vi "Valid Measurement Service Name.vi"(8 "error in":errorcluster, 11 "requested plugin name":string) -> (0 "error out":errorcluster, 3 "valid name?":bool)   [LabVIEW 2021, in "Migrator.lvlib"]
uses:
  Migrator.lvlib
  48953c88-0603-4c13-ba6a-df914321b09e.vi
  <vilib>/Comparison/Equal/Equal Functor/Equal Functor.lvclass
  Measurement Plugin Generator/_Editor/MeasurementService Editor.lvlib
panel:
  out "control chars":string
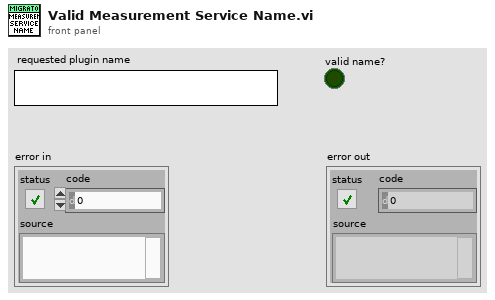
[diagram p1: front panel]
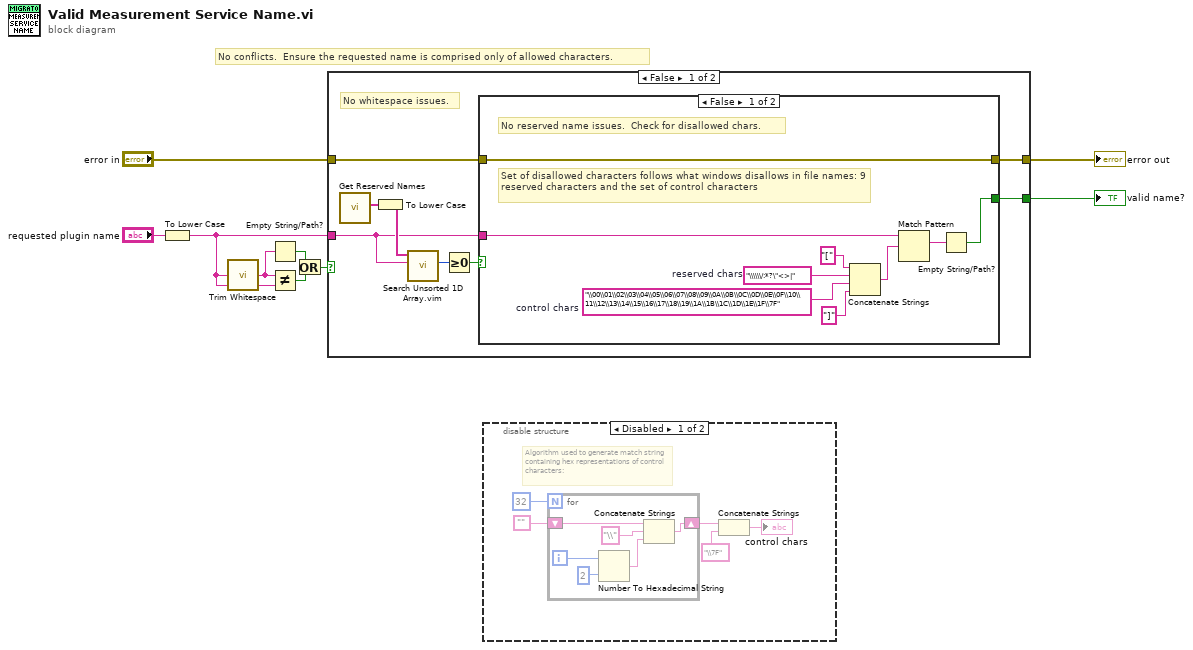
[diagram p0: block diagram]
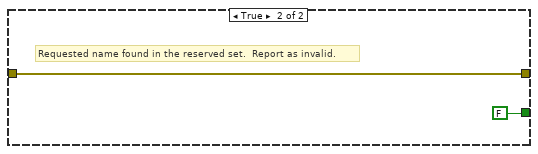
[diagram p2: hidden frame]
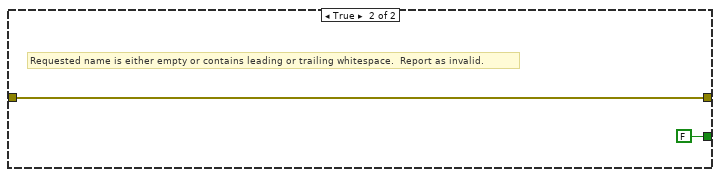
[diagram p3: hidden frame]
diagram:
  # "No conflicts.  Ensure the requested name is comprised only of allowed characters."
  n1 = To Lower Case(string="requested plugin name") -> (all lower case string=w5:string)
  n2 = call <vilib>:"Trim Whitespace.vi"("string"=w5) -> ("trimmed string"=w4:string)  [unwired: 1 in]
  n3 = Empty String/Path?(string/path=w4) -> (empty?=w2:bool)
  n4 = Not Equal?(x=w4, y=w5) -> (x != y?=w3:bool)
  n5 = Or(x=w2, y=w3) -> (x .or. y?=w1:bool)
  n6 = case shown="False" w1 {
    tunnel: w5 -> [w13 _]
    tunnel: "error in" -> [w17 w30]
    tunnel: [w16 w30] -> w7
    tunnel: [w10 FALSE ("Error if not Found (T)")] -> w6
    frame False {
      # "No whitespace issues."
      n7 = call "Get Reserved Names.vi"() -> ("reserved names"=w15:string[])  [unwired: 11 in]
      n8 = To Lower Case(string=w15) -> (all lower case string=w14:string[])
      n9 = call "Search Unsorted 1D Array.vim"("element"=w13, "unsorted 1D array"=w14) -> ("index of element"=w12:i32)  [unwired: 9 in]
      n10 = Greater Or Equal To 0?(x=w12) -> (x >= 0?=w11:bool)
      n11 = case shown="False" w11 {
        tunnel: w13 -> [w25 _]
        tunnel: w17 -> [w26 w28]
        tunnel: [w26 w28] -> w16
        tunnel: [w23 FALSE ("Error if not Found (T)")] -> w10
        frame False {
          w18 = "\\00\\01\\02\\03\\04\\05\\06\\07\\08\\09\\0A\\0B\\0C\\0D\\0E\\0F\\10\\11\\12\\13\\14\\15\\16\\17\\18\\19\\1A\\1B\\1C\\1D\\1E\\1F\\7F"  # control chars
          w22 = "\\\\\\/:*?\"<>|"  # reserved chars
          # "Set of disallowed characters follows what windows disallows in file names: 9 reserved characters and the set of control characters"
          # "No reserved name issues.  Check for disallowed chars."
          n12 = Concatenate Strings("[" ("string"), w22, w18, "]" ("string")) -> (w19:string)
          n13 = Match Pattern(string=w25, regular expression=w19) -> (match substring=w24:string)  [unwired: 1 in, 3 out]
          n14 = Empty String/Path?(string/path=w24) -> (empty?=w23:bool)
        }
        frame True {
          # "Requested name found in the reserved set.  Report as invalid."
        }
      }
    }
    frame True {
      # "Requested name is either empty or contains leading or trailing whitespace.  Report as invalid."
    }
  }
  "error out" <- w7
  "valid name?" <- w6
  n15 = disable-structure shown="Disabled" {
    frame Disabled {
      # "Algorithm used to generate match string containing hex representations of control characters:"
      n16 = for {
        N: 32 -> [_]
        shift-right: [w37] -> w33
        shift-left: "" -> [w36]
        i -> [w41]
        n17 = Number To Hexadecimal String(1:i16 2 ("width (-)"), 2:w41) -> (0:w39:string)
        n18 = Concatenate Strings(w36, "\\" ("string"), w39) -> (w37:string)
      }
      n19 = Concatenate Strings(w33, "\\7F") -> (→"control chars":string)
    }
    frame Enabled {
    }
  }
